vi "SSE.vi"(7 "LabVIEW Web Service Request":refnum<class "Web Request.lvclass">=refnum, 10 "variables":string, 11 "expId":string) -> ()   [LabVIEW 2014]
uses:
  <vilib>/wsapi/Web Request.lvclass
  Configuration/Global_Configurations.vi
  <vilib>/wsapi/class/subVIs/Write Integer Session Variable.vi
panel:
  out "expIndex":i32
  # "Use the Web Service Request input terminal to call the VIs on the Web Services palette. Do not remove it from the connector pane unless you don't need access to the palette."
  # "Each additional control wired to the connector pane will be available as an input in the URL. To include an indicator in terminal-mode output (the default setting), it must also be wired to the connector pane."
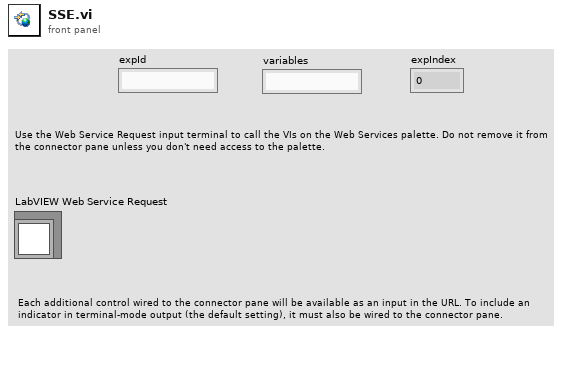
[diagram p1: front panel]
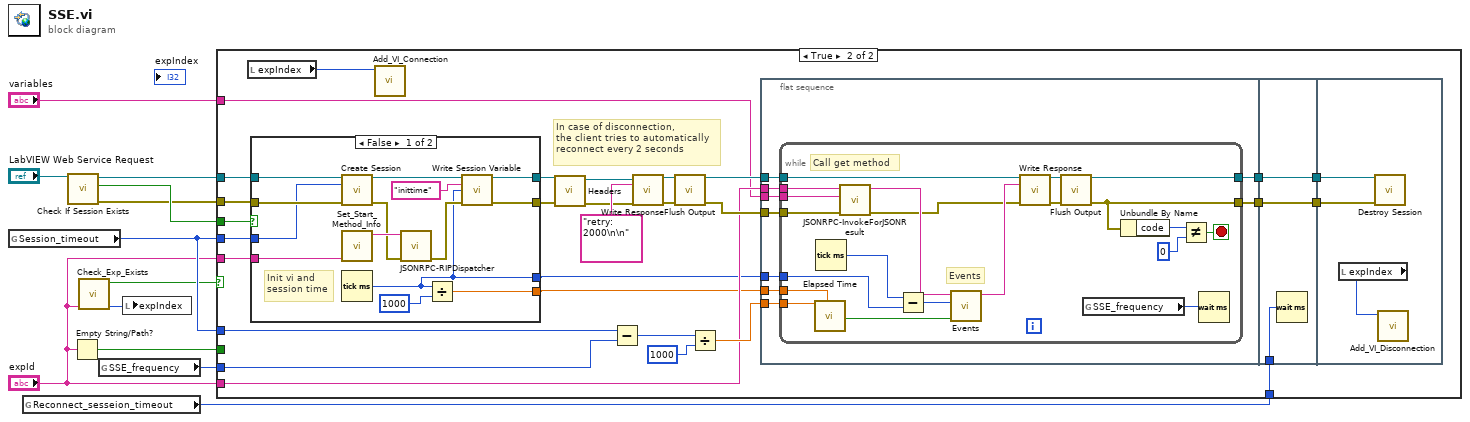
[diagram p0: block diagram]
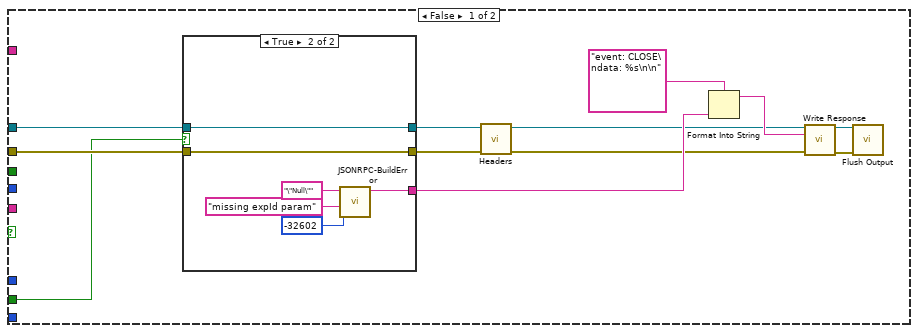
[diagram p2: hidden frame]
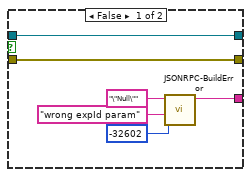
[diagram p3: hidden frame]
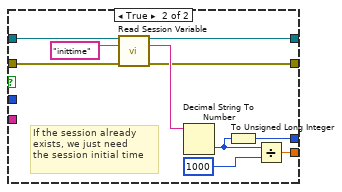
[diagram p4: hidden frame]
diagram:
  n1 = global read "Global_Configurations.vi" "Session_timeout"() -> (w9:u32)
  n2 = global read "Global_Configurations.vi" "Reconnect_sesseion_timeout"() -> (w10:u32)
  n3 = call <vilib>:"Check If Session Exists.vi"("LabVIEW Web Service Request"="LabVIEW Web Service Request") -> ("LabVIEW Web Service Request out"=w3:refnum<class "Web Request.lvclass">, "session exists?"=w7:bool, "error out"=w2:errorcluster)  [unwired: 12 in]
  n4 = Empty String/Path?(string/path="expId") -> (empty?=w5:bool)
  n5 = call "Check_Exp_Exists.vi"("expId"="expId") -> ("expIndex"=w1:i32, "exists"=w8:bool)  [unwired: 9 in]
  n6 = global read "Global_Configurations.vi" "SSE_frequency"() -> (w11:u32)
  n7 = local write "expIndex"(w1) -> ()
  n8 = case shown="True" w8 {
    tunnel: "expId" -> [_ w52]
    tunnel: w9 -> [_ w60]
    tunnel: w11 -> [_ w57]
    tunnel: w10 -> [_ w55]
    tunnel: w3 -> [w24 w54]
    tunnel: w2 -> [w23 w53]
    tunnel: "expId" -> [_ w49]
    tunnel: w7 -> [_ w48]
    tunnel: w9 -> [_ w47]
    tunnel: w5 -> [w22 _]
    tunnel: "variables" -> [_ w46]
    frame False {
      n9 = case shown="True" w22 {
        tunnel: w24 -> [w30 w32]
        tunnel: w23 -> [w29 w31]
        tunnel: [w25 w33] -> w17
        tunnel: [w30 w32] -> w16
        tunnel: [w29 w31] -> w15
        frame False {
          n10 = call "JSONRPC-BuildError.vi"("Message"="wrong expId param", "Code"=-32602, "ID"="\"Null\"") -> ("String"=w25:string)  [unwired: 8 in]
        }
        frame True {
          n11 = call "JSONRPC-BuildError.vi"("Message"="missing expId param", "Code"=-32602, "ID"="\"Null\"") -> ("String"=w33:string)  [unwired: 8 in]
        }
      }
      n12 = call "Headers.vi"("error in (no error)"=w15, "LabVIEW Web Service Request"=w16) -> ("error out"=w13:errorcluster, "LabVIEW Web Service Request out"=w14:refnum<class "Web Request.lvclass">)  [unwired: 8 in]
      n13 = Format Into String(format string="event: CLOSE\ndata: %s\n\n", w17) -> (resulting string=w21:string)  [unwired: 2 in, 1 out]
      n14 = call <vilib>:"Write Response.vi"("LabVIEW Web Service Request"=w14, "response string"=w21, "error in (no error)"=w13) -> ("LabVIEW Web Service Request out"=w19:refnum<class "Web Request.lvclass">, "error out"=w18:errorcluster)  [unwired: 11 in]
      n15 = call <vilib>:"Flush Output.vi"("LabVIEW Web Service Request"=w19, "error in (no error)"=w18) -> ()  [unwired: 12 in, 2 out]
    }
    frame True {
      # "In case of disconnection,\nthe client tries to automatically\nreconnect every 2 seconds"
      n16 = local read "expIndex"() -> (w41:i32)
      n17 = case shown="False" w48 {
        tunnel: w54 -> [w79 w87]
        tunnel: [w67 w80] -> w44
        tunnel: w53 -> [w78 w86]
        tunnel: [w66 w85] -> w45
        tunnel: w47 -> [w77 _]
        tunnel: w49 -> [w76 _]
        tunnel: [w68 w83] -> w50
        tunnel: [w69 w82] -> w51
        frame False {
          # "Init vi and \nsession time"
          n18 = call <vilib>:"Create Session.vi"("LabVIEW Web Service Request"=w79, "timeout (60000 msec)"=w77, "error in (no error)"=w78) -> ("LabVIEW Web Service Request out"=w72:refnum<class "Web Request.lvclass">, "error out"=w74:errorcluster)  [unwired: 10 in, 1 out]
          n19 = call "Set_Start_Method_Info.vi"("expId"=w76) -> ("String"=w75:string)  [unwired: 10 in]
          n20 = Tick Count (ms)() -> (millisecond timer value=w69:u32)
          n21 = call "JSONRPC-RIPDispatcher.vi"("error in"=w74, "input string"=w75) -> ("error out"=w71:errorcluster)  [unwired: 8 in, 1 out]
          n22 = Divide(x=w69, y=u32 1000) -> (x/y=w68:dbl)
          n23 = call-poly <vilib>:"Write Session Variable.vi"("LabVIEW Web Service Request"=w72, "key"="inittime", "value"=w69, "error in (no error)"=w71) -> ("LabVIEW Web Service Request out"=w67:refnum<class "Web Request.lvclass">, "error out"=w66:errorcluster)  [unwired: 8 in, 2 out]
        }
        frame True {
          # "If the session already exists, we just need \nthe session initial time"
          n24 = call <vilib>:"Read Session Variable.vi"("LabVIEW Web Service Request"=w87, "key"="inittime", "error in (no error)"=w86) -> ("LabVIEW Web Service Request out"=w80:refnum<class "Web Request.lvclass">, "value"=w89:string, "error out"=w85:errorcluster)  [unwired: 10 in]
          n25 = Decimal String To Number(string=w89) -> (number=w81:i32)  [unwired: 2 in, 1 out]
          n26 = To Unsigned Long Integer(number=w81) -> (unsigned 32bit integer=w82:u32)
          n27 = Divide(x=w81, y=u32 1000) -> (x/y=w83:dbl)
        }
      }
      n28 = call "Add_VI_Connection.vi"("expIndex"=w41) -> ()  [unwired: 11 in]
      n29 = call "Headers.vi"("error in (no error)"=w45, "LabVIEW Web Service Request"=w44) -> ("error out"=w42:errorcluster, "LabVIEW Web Service Request out"=w43:refnum<class "Web Request.lvclass">)  [unwired: 8 in]
      n30 = Subtract(x=w60, y=w57) -> (x-y=w56:u32)
      n31 = call <vilib>:"Write Response.vi"("LabVIEW Web Service Request"=w43, "response string"="retry: 2000\n\n", "error in (no error)"=w42) -> ("LabVIEW Web Service Request out"=w65:refnum<class "Web Request.lvclass">, "error out"=w64:errorcluster)  [unwired: 11 in]
      n32 = call <vilib>:"Flush Output.vi"("LabVIEW Web Service Request"=w65, "error in (no error)"=w64) -> ("LabVIEW Web Service Request out"=w63:refnum<class "Web Request.lvclass">, "error out"=w62:errorcluster)  [unwired: 12 in]
      n33 = Divide(x=w56, y=u32 1000) -> (x/y=w58:dbl)
      n34 = flat-sequence {
        tunnel: w63 -> [w98]
        tunnel: w62 -> [w97]
        tunnel: w52 -> [w96]
        tunnel: w50 -> [w95]
        tunnel: w58 -> [w94]
        tunnel: w51 -> [w93]
        tunnel: w46 -> [w92]
        tunnel: [w91] -> w39
        tunnel: [w90] -> w38
        tunnel: w55 -> [w122]
        tunnel: [w121] -> w40
        tunnel: w39 -> [w121]
        tunnel: w38 -> [w120]
        tunnel: [w120] -> w37
        tunnel: w40 -> [w124]
        tunnel: w37 -> [w123]
        frame #0 {
          n35 = while {
            tunnel: w98 -> [w108]
            tunnel: w97 -> [w113]
            tunnel: w96 -> [w114]
            tunnel: w95 -> [w105]
            tunnel: w94 -> [w107]
            tunnel: w93 -> [w103]
            tunnel: [w101] -> w91
            tunnel: [w100] -> w90
            tunnel: w92 -> [w99]
            stop <- w115 stop-if-true
            # "Events"
            # "Call get method"
            n36 = call "Elapsed Time"("Time Target (s)"=w107, "Set Start Time (s)"=w105) -> ("Time has Elapsed"=w106:bool)  [unwired: 10 in, 7 out]
            n37 = Tick Count (ms)() -> (millisecond timer value=w104:u32)
            n38 = call "JSONRPC-InvokeForJSONResult.vi"("error in"=w113, "variables"=w99, "expid"=w114) -> ("error out"=w109:errorcluster, "response"=w111:string)  [unwired: 7 in]
            n39 = Subtract(x=w104, y=w103) -> (x-y=w102:u32)
            n40 = call "Events.vi"("hearbeat"=w106, "time"=w102, "responsein"=w111) -> ("responseout"=w112:string)  [unwired: 8 in]
            n41 = call <vilib>:"Write Response.vi"("LabVIEW Web Service Request"=w108, "response string"=w112, "error in (no error)"=w109) -> ("LabVIEW Web Service Request out"=w118:refnum<class "Web Request.lvclass">, "error out"=w119:errorcluster)  [unwired: 11 in]
            n42 = call <vilib>:"Flush Output.vi"("LabVIEW Web Service Request"=w118, "error in (no error)"=w119) -> ("LabVIEW Web Service Request out"=w101:refnum<class "Web Request.lvclass">, "error out"=w100:errorcluster)  [unwired: 12 in]
            n43 = global read "Global_Configurations.vi" "SSE_frequency"() -> (w110:u32)
            n44 = Unbundle By Name(w100) -> ("code"=w117:i32)
            n45 = Not Equal?(x=w117, y=0) -> (x != y?=w115:bool)
            n46 = Wait (ms)(milliseconds to wait=w110) -> ()  [unwired: 1 out]
          }
        }
        frame #1 {
          n47 = Wait (ms)(milliseconds to wait=w122) -> ()  [unwired: 1 out]
        }
        frame #2 {
          n48 = local read "expIndex"() -> (w125:i32)
          n49 = call <vilib>:"Destroy Session.vi"("LabVIEW Web Service Request"=w124, "error in (no error)"=w123) -> ()  [unwired: 12 in, 2 out]
          n50 = call "Add_VI_Disconnection.vi"("expIndex"=w125) -> ()  [unwired: 11 in]
        }
      }
    }
  }
